vi "Write Task Factory CMD.vi"(8 "error in (no error)":errorcluster, 10 "Task Factory CMD":T1 caption="Enum 3", 11 "Task Factory MSG in":refnum<class "Task Factory MSG.lvclass">) -> (0 "error out":errorcluster, 3 "Task Factory MSG out":refnum<class "Task Factory MSG.lvclass">)   [LabVIEW 2024, in "Task Factory MSG.lvclass"]
uses:
  Task Factory MSG.lvclass
  Type Def/Task Factory CMD.ctl
  Task Factory MSG.lvclass/Task Factory MSG.ctl
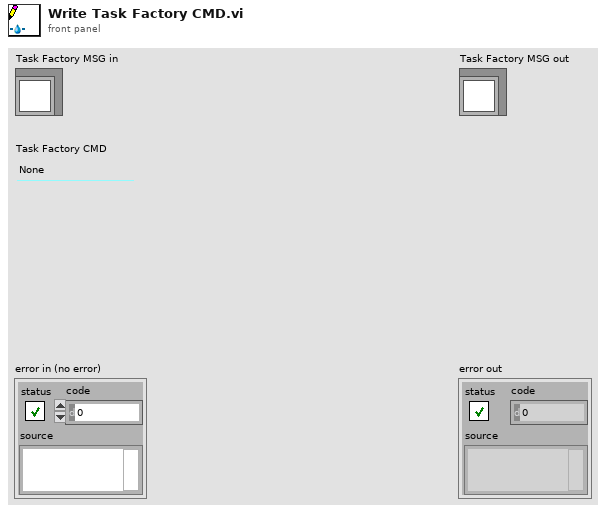
[diagram p1: front panel]
types:
  T1 = typedef "Task Factory CMD.ctl" = enum16{"None", "Generate Task"}
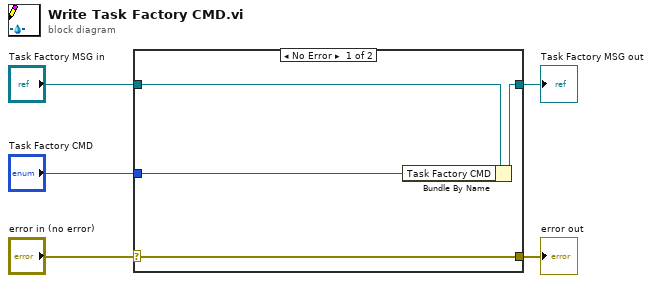
[diagram p0: block diagram]
diagram:
  n1 = case shown="No Error" "error in (no error)" {
    selector: "error in (no error)" -> [w9 w10]
    tunnel: [w9 w10] -> w4
    tunnel: [w7 w11] -> w2
    tunnel: "Task Factory MSG in" -> [w8 w11]
    tunnel: "Task Factory CMD" -> [w6 _]
    frame No Error {
      n2 = Bundle By Name(cluster=w8, "Task Factory CMD"=w6) -> (w7:refnum<class "Task Factory MSG.lvclass">)
    }
    frame Error {
    }
  }
  "error out" <- w4
  "Task Factory MSG out" <- w2
